vi "Drive PID.vi"(11 "Process Variable":dbl format="%.2f") -> (3 "Output":dbl format="%.2f")   [LabVIEW 2014]
uses:
  <vilib>/Rock Robotics/WPI/DriverStation/WPI_DriverStationRobotMode2.ctl
  <vilib>/addons/control/pid/pid.llb/PID (DBL).vi
  Begin/Global Variables.vi
  <vilib>/addons/control/pid/NI_PID_pid.lvlib
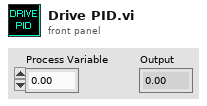
[diagram p1: front panel]
types:
  T1 = cluster{"proportional gain (Kc)":dbl, "integral time (Ti, min)":dbl, "derivative time (Td, min)":dbl}
  T2 = typedef "WPI_DriverStationRobotMode2.ctl" = enum16{"Autonomous Disabled", "Autonomous Enabled", "Teleop Disabled", "Teleop Enabled", "Disconnected", "Finish", "Test Disabled", "Test Enabled", "Emergency Stopped"}
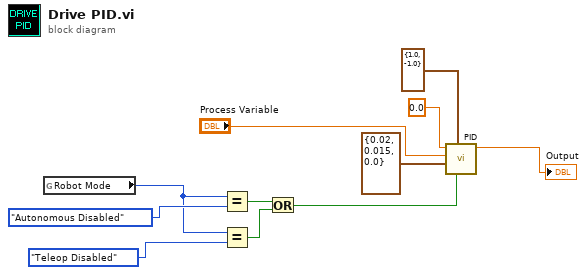
[diagram p0: block diagram]
diagram:
  n1 = global read "Global Variables.vi" "Robot Mode"() -> (w4:T2)
  n2 = Equal?(x=w4, y=WPI_DriverStationRobotMode2."Autonomous Disabled" ("Robot Mode")) -> (x = y?=w9:bool)
  n3 = Equal?(x=w4, y=WPI_DriverStationRobotMode2."Teleop Disabled" ("Robot Mode")) -> (x = y?=w8:bool)
  n4 = Or(x=w9, y=w8) -> (x .or. y?=w7:bool)
  n5 = call-poly <vilib>:"PID.vi"("reinitialize? (F)"=w7, "output range"=cluster{"output high":dbl, "output low":dbl} {"output high"=1.0, "output low"=-1.0}, "PID gains"=T1 {"proportional gain (Kc)"=0.02, "integral time (Ti, min)"=0.015, "derivative time (Td, min)"=0.0}, "process variable"="Process Variable", "setpoint"=0.0) -> ("output"=→"Output":dbl)  [unwired: 5 in, 1 out]
